vi "dvp Vi Get Analog Gain.vi"(10 "pAnalogGain":sgl, 11 "handle":u32) -> (2 "pAnalogGain out":sgl, 3 "function return":u32(ring))   [LabVIEW 2018, in "LabViewDVPCamera.lvlib"]
doc: "LabviewDvp2Api dvpStatus dvpViGetAnalogGain(dvpHandle handle, float *pAnalogGain);"
uses:
  LabViewDVPCamera.lvlib
  LabViewDVPCamera/LabViewDVPCamera.dll
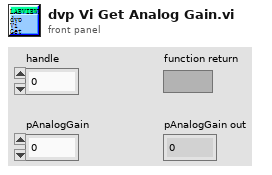
[diagram p1: front panel]
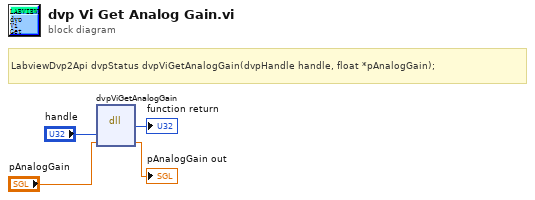
[diagram p0: block diagram]
diagram:
  # "LabviewDvp2Api dvpStatus dvpViGetAnalogGain(dvpHandle handle, float *pAnalogGain);"
  n1 = dll-call lib="C:/Program Files (x86)/DVP2 Labview cn 64/Sample/LabViewDVPCamera/LabViewDVPCamera.*" fn="dvpViGetAnalogGain"("handle"="handle", "pAnalogGain"="pAnalogGain") -> (→"function return":u32, "pAnalogGain"=→"pAnalogGain out":sgl)  [unwired: 4 in, 2 out]
